vi "updateChannelList.vi"(8 "error in (no error)":errorcluster, 11 "StaticOutputEditor in":refnum<class "StaticOutputEditor.lvclass">) -> (0 "error out":errorcluster, 3 "StaticOutputEditor out":refnum<class "StaticOutputEditor.lvclass">)   [LabVIEW 2011, in "Views.lvlib" / "ScriptEditor.lvlib" / "StaticOutputEditor.lvclass"]
uses:
  StaticOutputEditor.lvclass
  StaticOutputEditor.lvclass/StaticOutputEditor.ctl
panel:
  out "Array":string[](array[string])
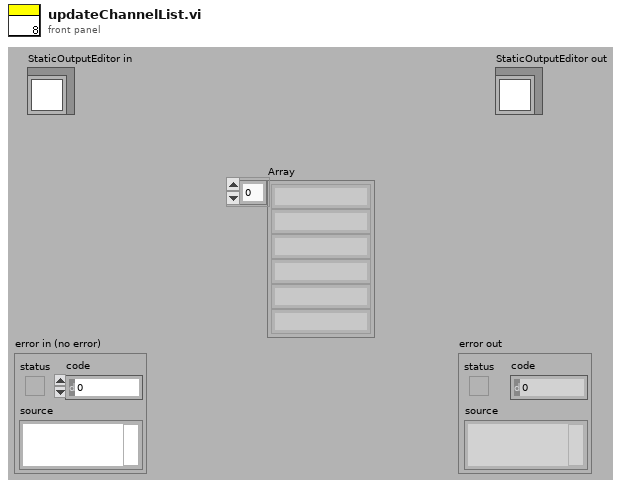
[diagram p1: front panel]
types:
  T1 = cluster{"channel":cluster{"calibration":cluster{"gradient":dbl, "offset":dbl}, "action":string, "safeState":string, "stateArray":string[], "units":string}, "channel Name":string, "channel address":string}[]
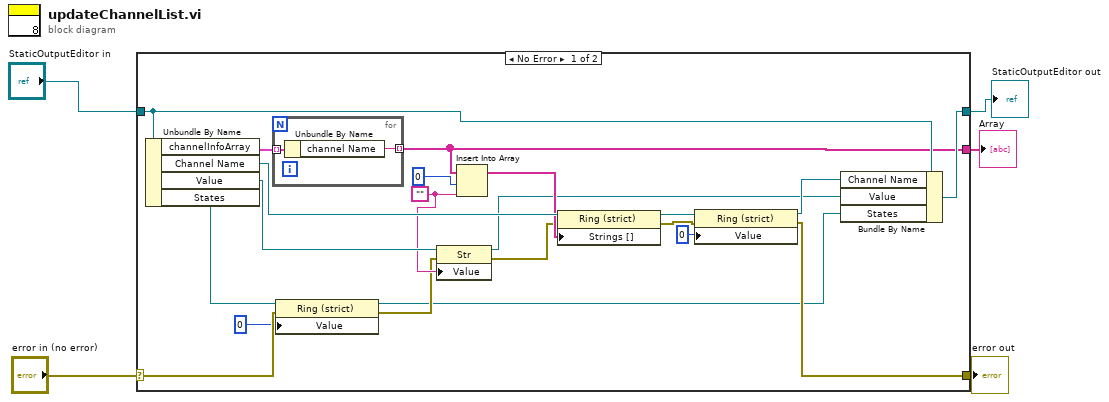
[diagram p0: block diagram]
diagram:
  n1 = case shown="No Error" "error in (no error)" {
    selector: "error in (no error)" -> [w12 w30]
    tunnel: [w15 w30] -> w4
    tunnel: [w21 w29] -> w2
    tunnel: "StaticOutputEditor in" -> [w22 w29]
    tunnel: [w20 _] -> w1
    frame No Error {
      w10 = ""
      n2 = Unbundle By Name(w22) -> ("channelInfoArray"=w26:T1, "Channel Name"=w25:refnum<vi>, "Value"=w14:refnum<vi>, "States"=w13:refnum<vi>)
      n3 = for {
        tunnel: w26 -> [w28] mode=indexing
        tunnel: [w27] -> w20 mode=indexing
        n4 = Unbundle By Name(w28) -> ("channel Name"=w27:string)
      }
      n5 = property class="Ring (strict)"(reference=w13, error in=w12, "Value"=0) -> (reference out=w8:refnum<vi>, error out=w9:errorcluster)
      n6 = property class="Str"(reference=w14, error in=w9, "Value"=w10) -> (reference out=w7:refnum<vi>, error out=w6:errorcluster)
      n7 = Insert Into Array(array=w20, index=0, new element=w10) -> (w23:string[])
      n8 = property class="Ring (strict)"(reference=w25, error in=w6, "Strings []"=w23) -> (reference out=w18:refnum<vi>, error out=w16:errorcluster)
      n9 = property class="Ring (strict)"(reference=w18, error in=w16, "Value"=u16 0) -> (reference out=w17:refnum<vi>, error out=w15:errorcluster)
      n10 = Bundle By Name(cluster=w22, "Channel Name"=w17, "Value"=w7, "States"=w8) -> (w21:refnum<class "StaticOutputEditor.lvclass">)
    }
    frame Error {
    }
  }
  "error out" <- w4
  "StaticOutputEditor out" <- w2
  "Array" <- w1
